vi "tmp_toml_file_read.vi"(8 "error in (no error)":errorcluster, 10 "operation (open or create)":T1(ring)=enum."open or create", 11 "path":path) -> (0 "error out":errorcluster, 3 "text":string)   [LabVIEW 2017]
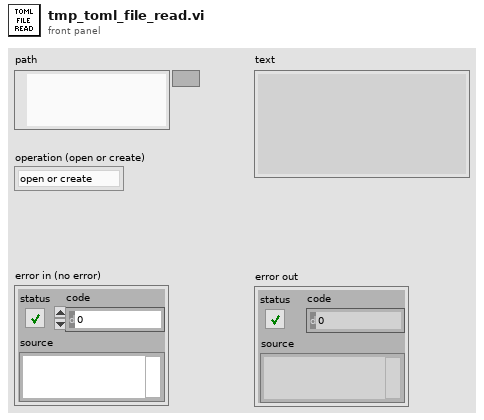
[diagram p1: front panel]
types:
  T1 = enum16{"open", "replace", "create", "open or create", "replace or create", "replace or create with confirmation"}
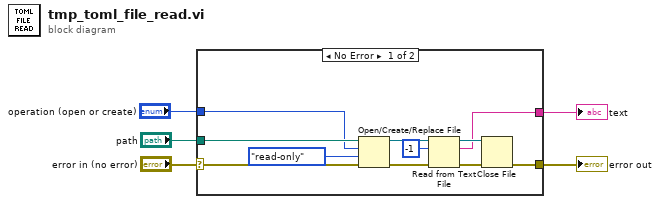
[diagram p0: block diagram]
diagram:
  n1 = case shown="No Error" "error in (no error)" {
    selector: "error in (no error)" -> [w16 w17]
    tunnel: "path" -> [w15 _]
    tunnel: [w10 _] -> w3
    tunnel: [w9 w17] -> w2
    tunnel: "operation (open or create)" -> [w7 _]
    frame No Error {
      n2 = Open/Create/Replace File(file path (use dialog)=w15, error in=w16, operation (0:open)=w7, access (0:read/write)=enum16{"read/write", "read-only", "write-only"}."read-only") -> (refnum out=w13:refnum<file>, error out=w14:errorcluster)  [unwired: 2 in, 1 out]
      n3 = Read from Text File(file (use dialog)=w13, count=-1, error in=w14) -> (refnum out=w11:refnum<file>, text=w10:string, error out=w12:errorcluster)  [unwired: 1 in, 1 out]
      n4 = Close File(refnum=w11, error in=w12) -> (error out=w9:errorcluster)  [unwired: 1 out]
    }
    frame Error {
    }
  }
  "error out" <- w2
  "text" <- w3
